vi "Read Attributes.vi"(11 "Fetch Room Details Msg":refnum<class "Fetch Room Details Msg.lvclass">) -> (2 "Payload":cluster{"Room No":string})   [LabVIEW 2023, in "Guest Manager UI.lvlib" / "Fetch Room Details Msg.lvclass"]
uses:
  Fetch Room Details Msg.lvclass
  Fetch Room Details Msg.lvclass/Fetch Room Details Msg.ctl
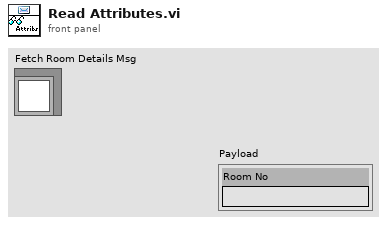
[diagram p1: front panel]
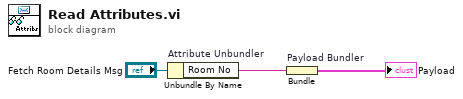
[diagram p0: block diagram]
diagram:
  n1 = Unbundle By Name "Attribute Unbundler"("Fetch Room Details Msg") -> ("Room No"=w1:string)
  n2 = Bundle "Payload Bundler"("Room No"=w1) -> (→"Payload":cluster{"Room No":string})  [unwired: 1 in]
